vi "Build Simple Skeleton Data.vi"(11 "data out":string) -> (0 "Kinect Outputs":T5, 1 "Skeleton Data":T6, 2 "NumPlayers":i8, 3 "Version String":string, 4 "Simple Joystick Info":T1(array[cluster]))   [LabVIEW 2011]
uses:
  <vilib>/addons/Kinect/SkeletonTrackState.ctl
  <vilib>/addons/Kinect/Vector4.ctl
  <vilib>/Rock Robotics/WPI/Joystick/WPI_JoystickDeviceDataRaw.ctl
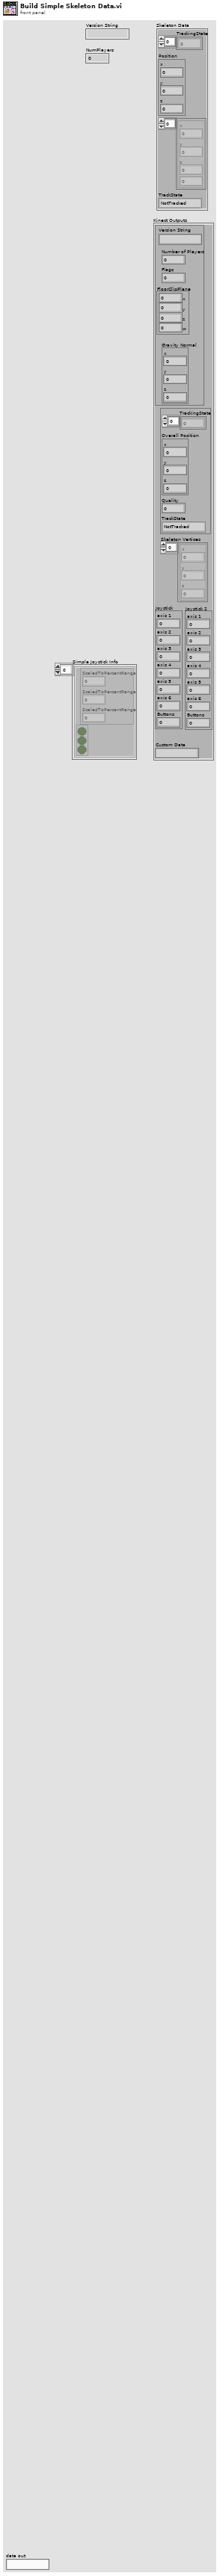
[diagram p1: front panel]
types:
  T1 = cluster{cluster{"ScaledToPercentRange":dbl, "ScaledToPercentRange":dbl, "ScaledToPercentRange":dbl}, cluster{bool, bool, bool}}[]
  T2 = typedef "Vector4.ctl" = cluster{"x":sgl, "y":sgl, "z":sgl, "w":sgl}
  T3 = typedef "SkeletonTrackState.ctl" = enum32{"NotTracked", "PositionOnly", "Tracked"}
  T4 = typedef "WPI_JoystickDeviceDataRaw.ctl" = cluster{"axis 1":i8, "axis 2":i8, "axis 3":i8, "axis 4":i8, "axis 5":i8, "axis 6":i8, "Buttons":u16}
  T5 = cluster{cluster{"Version String":string, "Number of Players":i8, "Flags":u32, "FloorClipPlane":T2, "Gravity Normal":cluster{"x":sgl, "y":sgl, "z":sgl}}, cluster{"TrackingState":u8[], "Overall Position":cluster{"x":sgl, "y":sgl, "z":sgl}, "Quality":u32, "TrackState":T3}, "Skeleton Vertices":cluster{"x":sgl, "y":sgl, "z":sgl}[], "Joystick":T4, "Joystick 2":T4, "Custom Data":string}
  T6 = cluster{"TrackingState":u8[], "Position":cluster{"x":sgl, "y":sgl, "z":sgl}, cluster{"x":sgl, "y":sgl, "z":sgl, sgl}[], "TrackState":T3}
  T7 = cluster{"size":u8, "tag":u8, "Version":cluster{"unsigned byte array[0]":u8, "unsigned byte array[1]":u8, "unsigned byte array[2]":u8, "unsigned byte array[3]":u8, "unsigned byte array[4]":u8, "unsigned byte array[5]":u8, "unsigned byte array[6]":u8, "unsigned byte array[7]":u8, "unsigned byte array[8]":u8, "unsigned byte array[9]":u8, "unsigned byte array[10]":u8}, "numPlayers":i8, "flags":u32, "floorClipPlane":T2, "Gravity Normal":cluster{"x":sgl, "y":sgl, "z":sgl}, "size":u8, "tag":u8, "Extra Data":cluster{"TrackingState":cluster{"TrackingState[0]":u8, "TrackingState[1]":u8, "TrackingState[2]":u8, "TrackingState[3]":u8, "TrackingState[4]":u8, "TrackingState[5]":u8, "TrackingState[6]":u8, "TrackingState[7]":u8, "TrackingState[8]":u8, "TrackingState[9]":u8, "TrackingState[10]":u8, "TrackingState[11]":u8, "TrackingState[12]":u8, "TrackingState[13]":u8, "TrackingState[14]":u8, "TrackingState[15]":u8, "TrackingState[16]":u8, "TrackingState[17]":u8, "TrackingState[18]":u8, "TrackingState[19]":u8}, "Position":cluster{"x":sgl, "y":sgl, "z":sgl}, "Quality":u32, "TrackState":T3}, "size":u8, "tag":u8, "Vertices":cluster{"Vertices[0]":cluster{"x":sgl, "y":sgl, "z":sgl}, "Vertices[1]":cluster{"x":sgl, "y":sgl, "z":sgl}, "Vertices[2]":cluster{"x":sgl, "y":sgl, "z":sgl}, "Vertices[3]":cluster{"x":sgl, "y":sgl, "z":sgl}, "Vertices[4]":cluster{"x":sgl, "y":sgl, "z":sgl}, "Vertices[5]":cluster{"x":sgl, "y":sgl, "z":sgl}, "Vertices[6]":cluster{"x":sgl, "y":sgl, "z":sgl}, "Vertices[7]":cluster{"x":sgl, "y":sgl, "z":sgl}, "Vertices[8]":cluster{"x":sgl, "y":sgl, "z":sgl}, "Vertices[9]":cluster{"x":sgl, "y":sgl, "z":sgl}, "Vertices[10]":cluster{"x":sgl, "y":sgl, "z":sgl}, "Vertices[11]":cluster{"x":sgl, "y":sgl, "z":sgl}, "Vertices[12]":cluster{"x":sgl, "y":sgl, "z":sgl}, "Vertices[13]":cluster{"x":sgl, "y":sgl, "z":sgl}, "Vertices[14]":cluster{"x":sgl, "y":sgl, "z":sgl}, "Vertices[15]":cluster{"x":sgl, "y":sgl, "z":sgl}, "Vertices[16]":cluster{"x":sgl, "y":sgl, "z":sgl}, "Vertices[17]":cluster{"x":sgl, "y":sgl, "z":sgl}, "Vertices[18]":cluster{"x":sgl, "y":sgl, "z":sgl}, "Vertices[19]":cluster{"x":sgl, "y":sgl, "z":sgl}}, "size":u8, "tag":u8, "Joystick":T4, "Joystick 2":T4, "size":u8, "tag":u8, "Custom Data":string}
  T8 = cluster{"unsigned byte array[0]":u8, "unsigned byte array[1]":u8, "unsigned byte array[2]":u8, "unsigned byte array[3]":u8, "unsigned byte array[4]":u8, "unsigned byte array[5]":u8, "unsigned byte array[6]":u8, "unsigned byte array[7]":u8, "unsigned byte array[8]":u8, "unsigned byte array[9]":u8, "unsigned byte array[10]":u8}
  T9 = cluster{"TrackingState[0]":u8, "TrackingState[1]":u8, "TrackingState[2]":u8, "TrackingState[3]":u8, "TrackingState[4]":u8, "TrackingState[5]":u8, "TrackingState[6]":u8, "TrackingState[7]":u8, "TrackingState[8]":u8, "TrackingState[9]":u8, "TrackingState[10]":u8, "TrackingState[11]":u8, "TrackingState[12]":u8, "TrackingState[13]":u8, "TrackingState[14]":u8, "TrackingState[15]":u8, "TrackingState[16]":u8, "TrackingState[17]":u8, "TrackingState[18]":u8, "TrackingState[19]":u8}
  T10 = cluster{"Vertices[0]":cluster{"x":sgl, "y":sgl, "z":sgl}, "Vertices[1]":cluster{"x":sgl, "y":sgl, "z":sgl}, "Vertices[2]":cluster{"x":sgl, "y":sgl, "z":sgl}, "Vertices[3]":cluster{"x":sgl, "y":sgl, "z":sgl}, "Vertices[4]":cluster{"x":sgl, "y":sgl, "z":sgl}, "Vertices[5]":cluster{"x":sgl, "y":sgl, "z":sgl}, "Vertices[6]":cluster{"x":sgl, "y":sgl, "z":sgl}, "Vertices[7]":cluster{"x":sgl, "y":sgl, "z":sgl}, "Vertices[8]":cluster{"x":sgl, "y":sgl, "z":sgl}, "Vertices[9]":cluster{"x":sgl, "y":sgl, "z":sgl}, "Vertices[10]":cluster{"x":sgl, "y":sgl, "z":sgl}, "Vertices[11]":cluster{"x":sgl, "y":sgl, "z":sgl}, "Vertices[12]":cluster{"x":sgl, "y":sgl, "z":sgl}, "Vertices[13]":cluster{"x":sgl, "y":sgl, "z":sgl}, "Vertices[14]":cluster{"x":sgl, "y":sgl, "z":sgl}, "Vertices[15]":cluster{"x":sgl, "y":sgl, "z":sgl}, "Vertices[16]":cluster{"x":sgl, "y":sgl, "z":sgl}, "Vertices[17]":cluster{"x":sgl, "y":sgl, "z":sgl}, "Vertices[18]":cluster{"x":sgl, "y":sgl, "z":sgl}, "Vertices[19]":cluster{"x":sgl, "y":sgl, "z":sgl}}
  T11 = cluster{"TrackingState":cluster{"TrackingState[0]":u8, "TrackingState[1]":u8, "TrackingState[2]":u8, "TrackingState[3]":u8, "TrackingState[4]":u8, "TrackingState[5]":u8, "TrackingState[6]":u8, "TrackingState[7]":u8, "TrackingState[8]":u8, "TrackingState[9]":u8, "TrackingState[10]":u8, "TrackingState[11]":u8, "TrackingState[12]":u8, "TrackingState[13]":u8, "TrackingState[14]":u8, "TrackingState[15]":u8, "TrackingState[16]":u8, "TrackingState[17]":u8, "TrackingState[18]":u8, "TrackingState[19]":u8}, "Position":cluster{"x":sgl, "y":sgl, "z":sgl}, "Quality":u32, "TrackState":T3}
  T12 = cluster{"ScaledToPercentRange":dbl, "ScaledToPercentRange":dbl, "ScaledToPercentRange":dbl}
  T13 = cluster{cluster{"ScaledToPercentRange":dbl, "ScaledToPercentRange":dbl, "ScaledToPercentRange":dbl}, cluster{bool, bool, bool}}
  T14 = cluster{"string":string, "numPlayers":i8, "flags":u32, "floorClipPlane":T2, "Gravity Normal":cluster{"x":sgl, "y":sgl, "z":sgl}}
  T15 = cluster{"TrackingState":u8[], "Position":cluster{"x":sgl, "y":sgl, "z":sgl}, "Quality":u32, "TrackState":T3}
  T16 = cluster{cluster{"string":string, "numPlayers":i8, "flags":u32, "floorClipPlane":T2, "Gravity Normal":cluster{"x":sgl, "y":sgl, "z":sgl}}, cluster{"TrackingState":u8[], "Position":cluster{"x":sgl, "y":sgl, "z":sgl}, "Quality":u32, "TrackState":T3}, "Vertices":cluster{"x":sgl, "y":sgl, "z":sgl}[], "Joystick":T4, "Joystick 2":T4, "Custom Data":string}
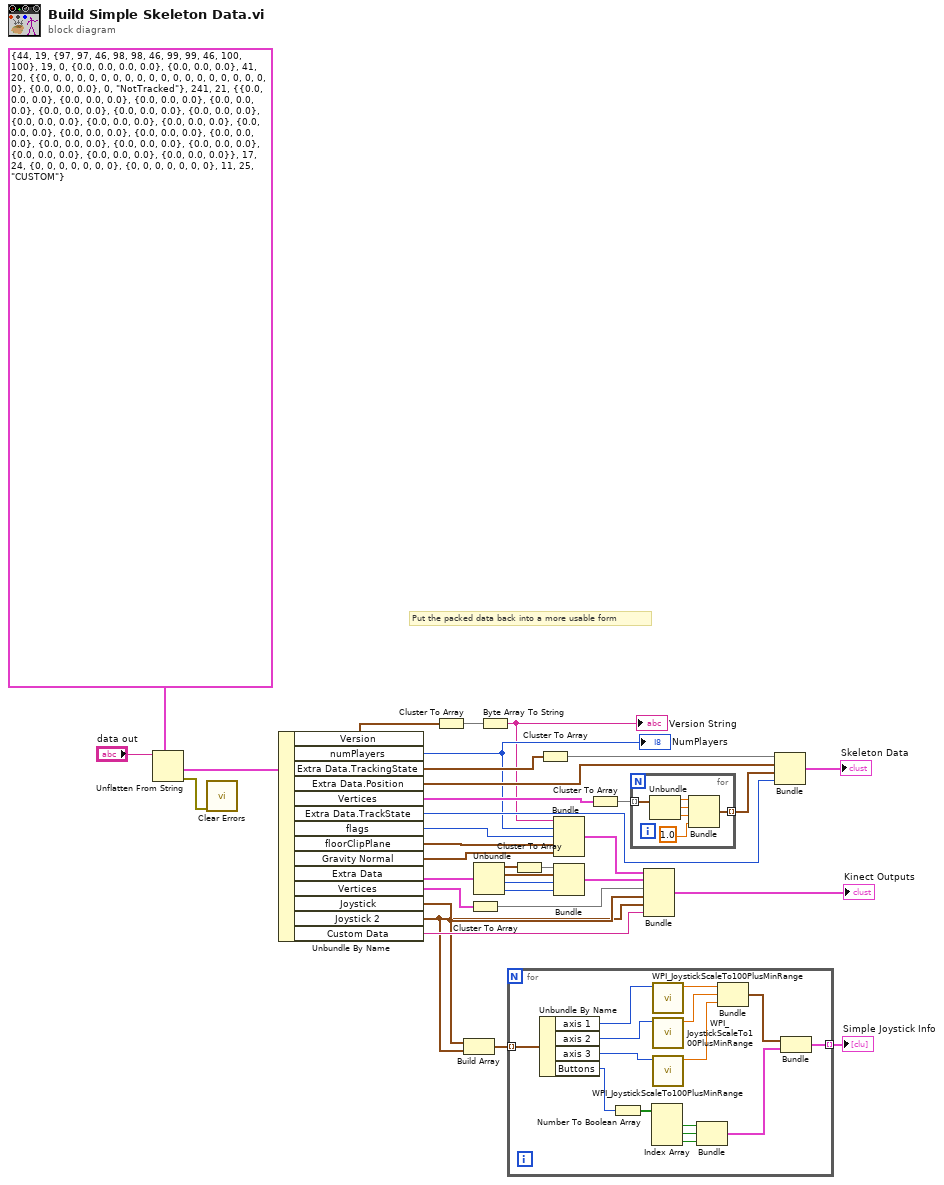
[diagram p0: block diagram]
diagram:
  # "Put the packed data back into a more usable form"
  n1 = Unflatten From String(type=T7 {"size"=44, "tag"=19, "Version"={"unsigned byte array[0]"=97, "unsigned byte array[1]"=97, "unsigned byte array[2]"=46, "unsigned byte array[3]"=98, "unsigned byte array[4]"=98, "unsigned byte array[5]"=46, "unsigned byte array[6]"=99, "unsigned byte array[7]"=99, "unsigned byte array[8]"=46, "unsigned byte array[9]"=100, "unsigned byte array[10]"=100}, "numPlayers"=19, "flags"=0, "floorClipPlane"={"x"=0.0, "y"=0.0, "z"=0.0, "w"=0.0}, "Gravity Normal"={"x"=0.0, "y"=0.0, "z"=0.0}, "size"=41, "tag"=20, "Extra Data"={"TrackingState"={"TrackingState[0]"=0, "TrackingState[1]"=0, "TrackingState[2]"=0, "TrackingState[3]"=0, "TrackingState[4]"=0, "TrackingState[5]"=0, "TrackingState[6]"=0, "TrackingState[7]"=0, "TrackingState[8]"=0, "TrackingState[9]"=0, "TrackingState[10]"=0, "TrackingState[11]"=0, "TrackingState[12]"=0, "TrackingState[13]"=0, "TrackingState[14]"=0, "TrackingState[15]"=0, "TrackingState[16]"=0, "TrackingState[17]"=0, "TrackingState[18]"=0, "TrackingState[19]"=0}, "Position"={"x"=0.0, "y"=0.0, "z"=0.0}, "Quality"=0, "TrackState"=enum."NotTracked"}, "size"=241, "tag"=21, "Vertices"={"Vertices[0]"={"x"=0.0, "y"=0.0, "z"=0.0}, "Vertices[1]"={"x"=0.0, "y"=0.0, "z"=0.0}, "Vertices[2]"={"x"=0.0, "y"=0.0, "z"=0.0}, "Vertices[3]"={"x"=0.0, "y"=0.0, "z"=0.0}, "Vertices[4]"={"x"=0.0, "y"=0.0, "z"=0.0}, "Vertices[5]"={"x"=0.0, "y"=0.0, "z"=0.0}, "Vertices[6]"={"x"=0.0, "y"=0.0, "z"=0.0}, "Vertices[7]"={"x"=0.0, "y"=0.0, "z"=0.0}, "Vertices[8]"={"x"=0.0, "y"=0.0, "z"=0.0}, "Vertices[9]"={"x"=0.0, "y"=0.0, "z"=0.0}, "Vertices[10]"={"x"=0.0, "y"=0.0, "z"=0.0}, "Vertices[11]"={"x"=0.0, "y"=0.0, "z"=0.0}, "Vertices[12]"={"x"=0.0, "y"=0.0, "z"=0.0}, "Vertices[13]"={"x"=0.0, "y"=0.0, "z"=0.0}, "Vertices[14]"={"x"=0.0, "y"=0.0, "z"=0.0}, "Vertices[15]"={"x"=0.0, "y"=0.0, "z"=0.0}, "Vertices[16]"={"x"=0.0, "y"=0.0, "z"=0.0}, "Vertices[17]"={"x"=0.0, "y"=0.0, "z"=0.0}, "Vertices[18]"={"x"=0.0, "y"=0.0, "z"=0.0}, "Vertices[19]"={"x"=0.0, "y"=0.0, "z"=0.0}}, "size"=17, "tag"=24, "Joystick"={"axis 1"=0, "axis 2"=0, "axis 3"=0, "axis 4"=0, "axis 5"=0, "axis 6"=0, "Buttons"=0}, "Joystick 2"={"axis 1"=0, "axis 2"=0, "axis 3"=0, "axis 4"=0, "axis 5"=0, "axis 6"=0, "Buttons"=0}, "size"=11, "tag"=25, "Custom Data"="CUSTOM"} ("output data"), binary string="data out") -> (value=w26:T7, error out=w23:errorcluster)  [unwired: 1 in, 3 out]
  n2 = call <vilib>:"Clear Errors.vi"("error in (no error)"=w23) -> ()  [unwired: 6 in, 1 out]
  n3 = Unbundle By Name(w26) -> ("Version"=w22:T8, "numPlayers"=w21:i8, "Extra Data.TrackingState"=w28:T9, "Extra Data.Position"=w34:cluster{"x":sgl, "y":sgl, "z":sgl}, "Vertices"=w33:T10, "Extra Data.TrackState"=w35:T3, "flags"=w20:u32, "floorClipPlane"=w19:T2, "Gravity Normal"=w18:cluster{"x":sgl, "y":sgl, "z":sgl}, "Extra Data"=w16:T11, "Vertices"=w9:T10, "Joystick"=w4:T4, "Joystick 2"=w2:T4, "Custom Data"=w5:string)
  "NumPlayers" <- w21
  n4 = Cluster To Array(cluster=w22) -> (array=w27:u8[])
  n5 = Build Array(w4, w2) -> (w3:T4[])
  n6 = Cluster To Array(cluster=w9) -> (array=w8:cluster{"x":sgl, "y":sgl, "z":sgl}[])
  n7 = Unbundle(w16) -> ("TrackingState"=w15:T9, "Position"=w13:cluster{"x":sgl, "y":sgl, "z":sgl}, "Quality"=w12:u32, "TrackState"=w11:T3)
  n8 = Byte Array To String(unsigned byte array=w27) -> (string=w6:string)
  "Version String" <- w6
  n9 = for {
    tunnel: w3 -> [w50] mode=indexing
    tunnel: [w36] -> w1 mode=indexing
    n10 = Unbundle By Name(w50) -> ("axis 1"=w44:i8, "axis 2"=w42:i8, "axis 3"=w41:i8, "Buttons"=w48:u16)
    n11 = Number To Boolean Array(number=w48) -> (Boolean array=w49:bool[])
    n12 = Index Array(array=w49) -> (element #1=w45:bool, element #2=w46:bool, element #3=w47:bool)  [unwired: 3 in]
    n13 = call <vilib>:"WPI_JoystickScaleTo100PlusMinRange.vi"("RawValue"=w44) -> ("ScaledToPercentRange"=w43:dbl)  [unwired: 1 in, 9 out]
    n14 = call <vilib>:"WPI_JoystickScaleTo100PlusMinRange.vi"("RawValue"=w42) -> ("ScaledToPercentRange"=w40:dbl)  [unwired: 1 in, 9 out]
    n15 = call <vilib>:"WPI_JoystickScaleTo100PlusMinRange.vi"("RawValue"=w41) -> ("ScaledToPercentRange"=w39:dbl)  [unwired: 1 in, 9 out]
    n16 = Bundle(w45, w46, w47) -> (w37:cluster{bool, bool, bool})  [unwired: 1 in]
    n17 = Bundle("ScaledToPercentRange"=w43, "ScaledToPercentRange"=w40, "ScaledToPercentRange"=w39) -> (w38:T12)  [unwired: 1 in]
    n18 = Bundle(w38, w37) -> (w36:T13)  [unwired: 1 in]
  }
  "Simple Joystick Info" <- w1
  n19 = Cluster To Array(cluster=w15) -> (array=w14:u8[])
  n20 = Cluster To Array(cluster=w28) -> (array=w30:u8[])
  n21 = Bundle("string"=w6, "numPlayers"=w21, "flags"=w20, "floorClipPlane"=w19, "Gravity Normal"=w18) -> (w17:T14)  [unwired: 1 in]
  n22 = Bundle("TrackingState"=w14, "Position"=w13, "Quality"=w12, "TrackState"=w11) -> (w10:T15)  [unwired: 1 in]
  n23 = Cluster To Array(cluster=w33) -> (array=w31:cluster{"x":sgl, "y":sgl, "z":sgl}[])
  n24 = for {
    tunnel: w31 -> [w56] mode=indexing
    tunnel: [w51] -> w32 mode=indexing
    n25 = Unbundle(w56) -> ("x"=w52:sgl, "y"=w53:sgl, "z"=w54:sgl)
    n26 = Bundle("x"=w52, "y"=w53, "z"=w54, sgl 1.0) -> (w51:cluster{"x":sgl, "y":sgl, "z":sgl, sgl})  [unwired: 1 in]
  }
  n27 = Bundle(w17, w10, "Vertices"=w8, "Joystick"=w4, "Joystick 2"=w2, "Custom Data"=w5) -> (→"Kinect Outputs":T16)  [unwired: 1 in]
  n28 = Bundle("TrackingState"=w30, "Position"=w34, w32, "TrackState"=w35) -> (→"Skeleton Data":T6)  [unwired: 1 in]
